vi "Ejercicio_3_1.vi"() -> ()   [LabVIEW 2020]
uses:
  <vilib>/numeric/Random Number (Range) DBL.vi
panel:
  out "min value":dbl
  out "max value":dbl
  out "Gráfica comparativa":dbl[][](graph)
  out "EMA":dbl[](graph)
  out "EMA":dbl[](array[numeric])
  out "appended array":dbl[][](array[numeric])
  out "F°":dbl[](array[numeric])
  out "Datos obtenidos":dbl(graph)
  out "C°":dbl[](array[numeric])
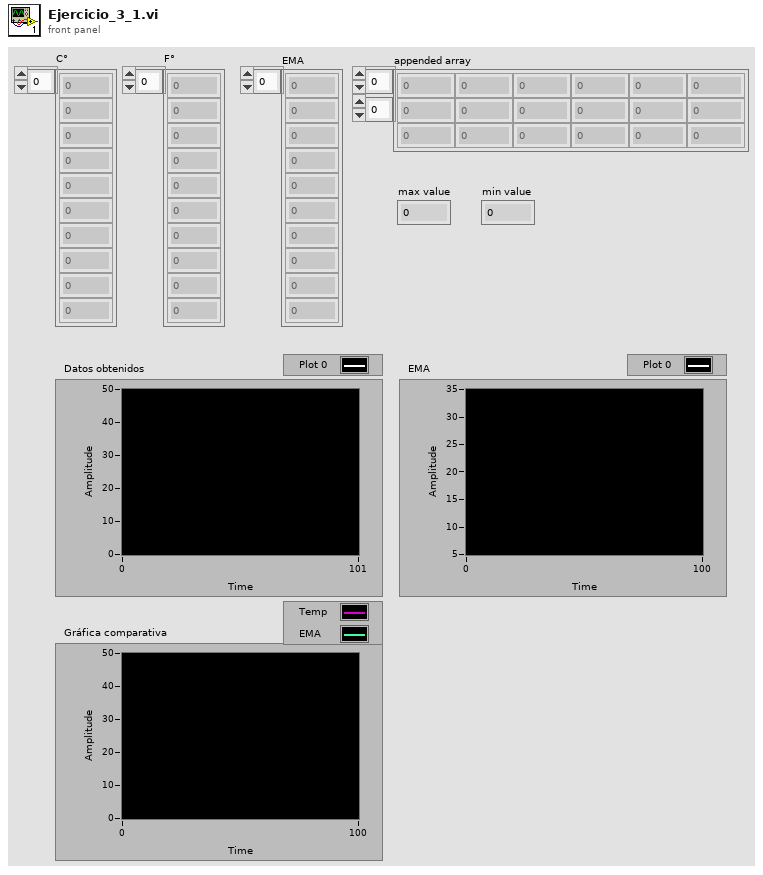
[diagram p1: front panel]
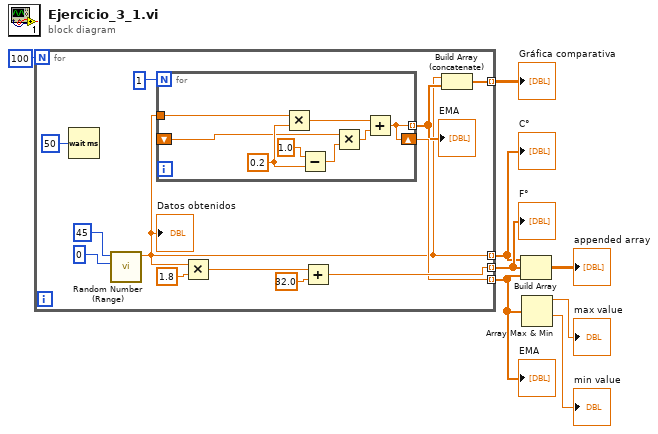
[diagram p0: block diagram]
diagram:
  n1 = for {
    N: 100 -> [_]
    tunnel: [w11] -> w5 mode=indexing
    tunnel: [w15] -> w7 mode=indexing
    tunnel: [w13] -> w4 mode=indexing
    tunnel: [w10] -> w1 mode=indexing
    n2 = Wait (ms)(milliseconds to wait=u32 50) -> ()  [unwired: 1 out]
    n3 = call-poly <vilib>:"Random Number (Range).vi"("lower bound (0)"=u64 0, "upper bound (100)"=u64 45) -> ("number"=w11:dbl)  [unwired: 9 in]
    "Datos obtenidos" <- w11
    n4 = for {
      N: 1 -> [_]
      tunnel: w11 -> [w23]
      shift-right: [w21] -> w13
      shift-left: _ -> [w22]
      tunnel: [w21] -> w12 mode=indexing
      w25 = 0.2 ("y")
      n5 = Multiply(x=w23, y=w25) -> (x*y=w28:dbl)
      n6 = Subtract(x=1.0, y=w25) -> (x-y=w27:dbl)
      n7 = Multiply(x=w22, y=w27) -> (x*y=w24:dbl)
      n8 = Add(x=w28, y=w24) -> (x+y=w21:dbl)
    }
    "EMA" <- w12
    n9 = Multiply(x=w11, y=1.8) -> (x*y=w20:dbl)
    n10 = Add(x=w20, y=32.0) -> (x+y=w15:dbl)
    n11 = Build Array (concatenate)(w11, w12) -> (w10:dbl[])
  }
  "C°" <- w5
  "F°" <- w7
  "EMA" <- w4
  "Gráfica comparativa" <- w1
  n12 = Build Array(w5, w7, w4) -> (→"appended array":dbl[][])
  n13 = Array Max & Min(array=w4) -> (max value=→"max value":dbl, min value=→"min value":dbl)  [unwired: 2 out]
